vi "Idle.vi"(8 "error in (no error)":errorcluster, 11 "Shutter in":refnum<class "Shutter.lvclass">) -> (0 "error out":errorcluster, 2 "State":T1=enum."Wait", 3 "Shutter out":refnum<class "Shutter.lvclass">)   [LabVIEW 2016, in "Shutter.lvclass"]
uses:
  Shutter.lvclass
  Controls/Shutter States.ctl
  Shutter.lvclass/Shutter.ctl
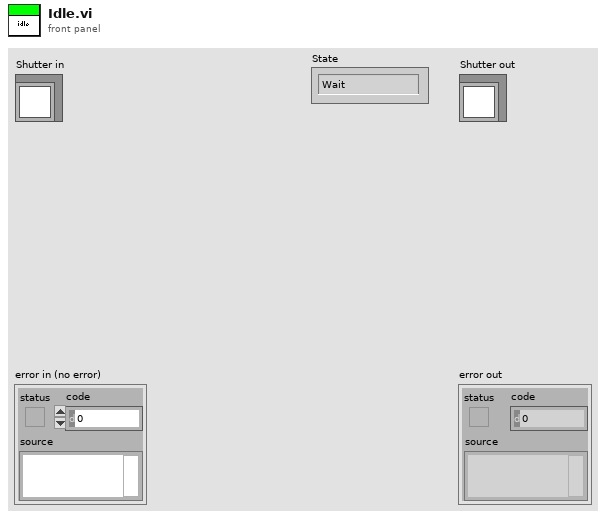
[diagram p1: front panel]
types:
  T1 = typedef "Shutter States.ctl" = enum16{"Open", "Close", "Wait", "Off", "Arm", "Idle"}
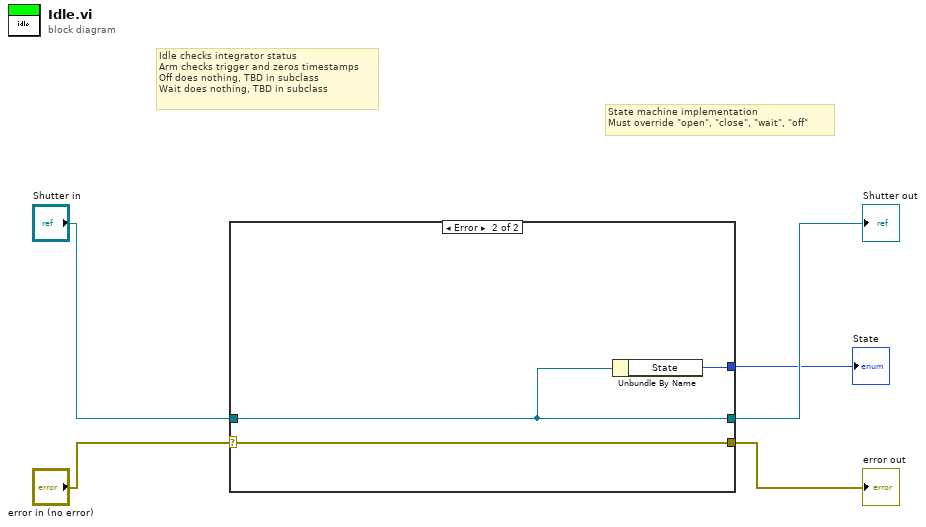
[diagram p0: block diagram]
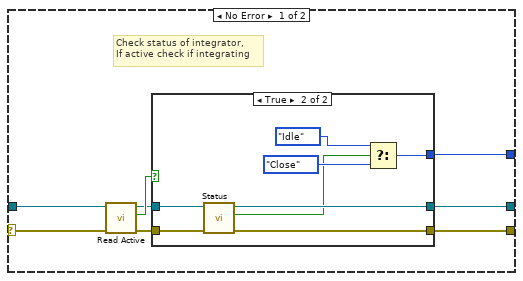
[diagram p2: hidden frame]
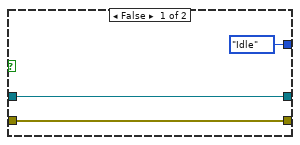
[diagram p3: hidden frame]
diagram:
  # "Idle checks integrator status \nArm checks trigger and zeros timestamps\nOff does nothing, TBD in subclass\nWait does nothing, TBD in subclass"
  # "State machine implementation\nMust override \"open\", \"close\", \"wait\", \"off\""
  n1 = case shown="Error" "error in (no error)" {
    selector: "error in (no error)" -> [w7 w27]
    tunnel: "Shutter in" -> [w13 w26]
    tunnel: [w12 w26] -> w4
    tunnel: [w11 w27] -> w3
    tunnel: [w6 w25] -> w1
    frame No Error {
      # "Check status of integrator,\nIf active check if integrating"
      n2 = call-dynamic "Read Active.vi"("error in (no error)"=w7, "Integrator in"=w13) -> ("error out"=w8:errorcluster, "Active"=w10:bool, "Integrator out"=w9:refnum<class "Shutter.lvclass">)  [unwired: 7 in]
      n3 = case shown="True" w10 {
        tunnel: [w15 w24] -> w12
        tunnel: [w16 w23] -> w11
        tunnel: w9 -> [w15 w20]
        tunnel: w8 -> [w16 w19]
        tunnel: [Shutter_States."Idle" ("f") w17] -> w6
        frame False {
        }
        frame True {
          n4 = call-dynamic "Status.vi"("error in (no error)"=w19, "Integrator in"=w20) -> ("error out"=w23:errorcluster, "Integrating"=w18:bool, "Integrator out"=w24:refnum<class "Shutter.lvclass">)  [unwired: 7 in]
          n5 = Select(t=Shutter_States."Idle" ("f"), s=w18, f=Shutter_States."Close") -> (s? t:f=w17:T1)
        }
      }
    }
    frame Error {
      n6 = Unbundle By Name(w26) -> ("State"=w25:T1)
    }
  }
  "error out" <- w3
  "Shutter out" <- w4
  "State" <- w1
